vi "Replace System.vi"(8 "error in (no error)":errorcluster, 10 "BME_DG_System":refnum<class "BME_DG_System.lvclass">, 11 "SystemsIn":refnum<class "BME_DG_System.lvclass">[](array[class])) -> (0 "error out":errorcluster, 3 "SystemsOut":refnum<class "BME_DG_System.lvclass">[](array[class]))   [LabVIEW 2009, in "POLARIS BME DG.lvlib" / "BME_DG_System.lvclass"]
uses:
  BME_DG_System.lvclass
  BME_DG_System.lvclass/BME_DG_System.ctl
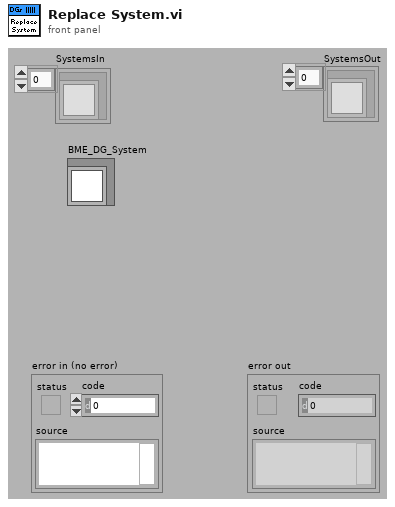
[diagram p1: front panel]
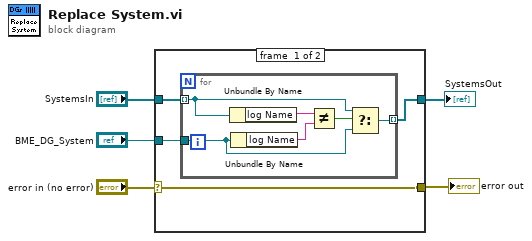
[diagram p0: block diagram]
diagram:
  n1 = case shown="No Error" "error in (no error)" {
    selector: "error in (no error)" -> [w6 w16]
    tunnel: "SystemsIn" -> [w9 w17]
    tunnel: "BME_DG_System" -> [w8 _]
    tunnel: [w7 w17] -> w2
    tunnel: [w6 w16] -> w1
    frame #0 {
      n2 = for {
        tunnel: w9 -> [w12] mode=indexing
        tunnel: w8 -> [w11]
        tunnel: [w10] -> w7 mode=indexing
        n3 = Unbundle By Name(w12) -> ("log Name"=w15:string)
        n4 = Unbundle By Name(w11) -> ("log Name"=w14:string)
        n5 = Not Equal?(x=w15, y=w14) -> (x != y?=w13:bool)
        n6 = Select(t=w12, s=w13, f=w11) -> (s? t:f=w10:refnum<class "BME_DG_System.lvclass">)
      }
    }
    frame #1 {
    }
  }
  "error out" <- w1
  "SystemsOut" <- w2
